vi "Sequence-UserAction.vi"(8 "error in (no error)":errorcluster, 10 "UserAction":T1=enum."Pause") -> (0 "error out":errorcluster)   [LabVIEW 2016]
uses:
  Sequence.UserAction.ctl
  Sequence.Action.ctl
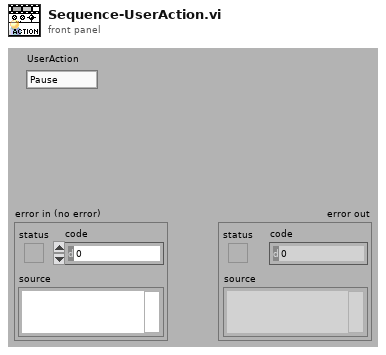
[diagram p1: front panel]
types:
  T1 = typedef "Sequence.UserAction.ctl" = enum16{"-", "Stop", "Pause", "Continue", "Next"}
  T2 = typedef "Sequence.Action.ctl" = enum32{"idle", "constructor", "destructor", "--- Sequence ---", "Abort", "Init", "Select", "Start", "Work.Run", "Work.AirON", "Work.LaserON", "Work.Done", "Process.Run", "Process.Engine", "Process.Pause", "Process.DoorLock", "Process.Wait4Container", "Process.Wait1", "Process.Wait2", "Process.Continue", "Process.Done", "Home.Run", "Home.AirON", "Home.TablePos", "Home.MoveServo", "Home.LaserOFF", "Home.AirOFF", "Home.Done", "User.Action", "User.Data", "Status.Clear"}
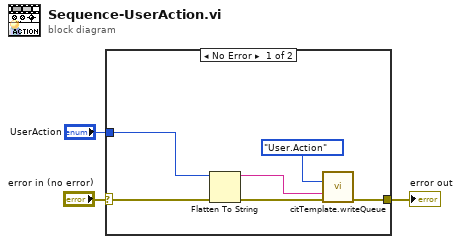
[diagram p0: block diagram]
diagram:
  n1 = case shown="No Error" "error in (no error)" {
    selector: "error in (no error)" -> [w8 w10]
    tunnel: [w9 w10] -> w2
    tunnel: "UserAction" -> [w5 _]
    frame No Error {
      n2 = Flatten To String(anything=w5, error in (no error)=w8) -> (data string=w4:string, error out=w6:errorcluster)  [unwired: 2 in, 1 out]
      n3 = call "citTemplate.writeQueue.vi"("event in (if not connected:all statemachine with data event)"=Sequence.Action."User.Action" ("Action"), "data in"=w4, "error in (no error)"=w6) -> ("error out"=w9:errorcluster)  [unwired: 12 in]
    }
    frame Error {
    }
  }
  "error out" <- w2
